vi "Load Image From Memory (Core).vi"(8 "error in (no error)":errorcluster, 9 "Transparency Threshold (127)":u8=127, 11 "Encoded Image":u8[](array[numeric])) -> (0 "error out":errorcluster, 2 "Image":T1)   [LabVIEW 2020, in "G-Image.lvlib"]
doc: "Decodes the byte array to a LabVIEW picture."
uses:
  G-Image.lvlib
  <vilib>/picture/picture.llb/imagedata.ctl
  <vilib>/Utility/file.llb/Application Directory.vi
  <vilib>/Utility/error.llb/Error Cluster From Error Code.vi
  lib/g_image_32.dll
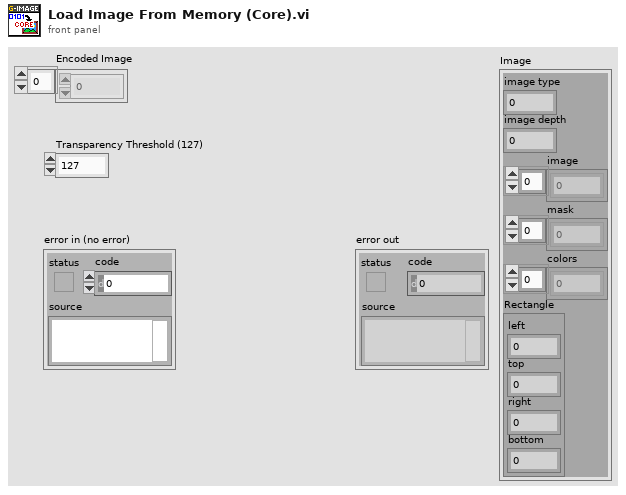
[diagram p1: front panel]
types:
  T1 = typedef "imagedata.ctl" = cluster{"image type":i32, "image depth":i32, "image":u8[], "mask":u8[], "colors":u32[], "Rectangle":cluster{"left":i16, "top":i16, "right":i16, "bottom":i16}}
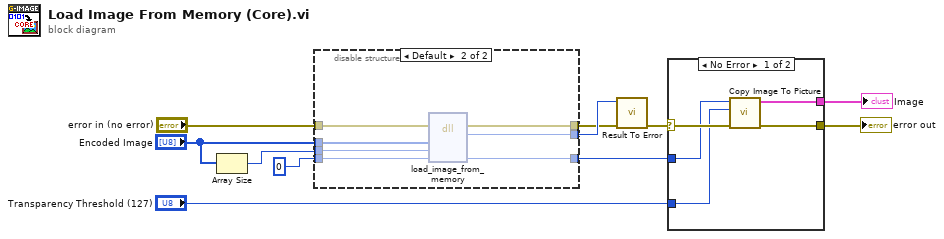
[diagram p0: block diagram]
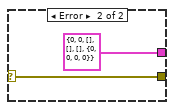
[diagram p2: hidden frame]
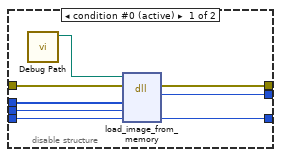
[diagram p3: hidden frame]
diagram:
  n1 = Array Size(array="Encoded Image") -> (size(s)=w2:i32)
  n2 = disable-structure shown="Default" {
    disable-tunnel: [w18 w26] -> w8
    disable-tunnel: "error in (no error)" -> [w17 w25]
    disable-tunnel: "Encoded Image" -> [w16 w24]
    disable-tunnel: [w15 w23] -> w9
    disable-tunnel: [w14 w21] -> w5
    disable-tunnel: i64 0 ("count") -> [w13 w22]
    disable-tunnel: w2 -> [w12 w20]
    frame condition #0 (active) {
      n3 = call "Debug Path.vi"() -> ("Debug Path"=w19:path)  [unwired: 11 in]
      n4 = dll-call lib="?" fn="load_image_from_memory"(path in=w19, error in=w17, "encoded_image"=w16, "encoded_image_size"=w12, "image_out"=w13) -> (error out=w18:errorcluster, "result"=w15:i32, "image_out"=w14:i64)  [unwired: 3 in, 1 out]
    }
    frame condition #1 {
      n5 = dll-call lib="C:/github/dataflowg/g-image/src/LabVIEW/G-Image/lib/g_image_*.*" fn="load_image_from_memory"(error in=w25, "encoded_image"=w24, "encoded_image_count"=w20, "image_out"=w22) -> (error out=w26:errorcluster, "result"=w23:i32, "image_out"=w21:i64)  [unwired: 4 in, 1 out]
    }
  }
  n6 = call "Result To Error.vi"("error in (no error)"=w8, "Result Code"=w9) -> ("error out"=w7:errorcluster)  [unwired: 9 in]
  n7 = case shown="No Error" w7 {
    selector: w7 -> [w31 w33]
    tunnel: [w29 w33] -> w11
    tunnel: w5 -> [w30 _]
    tunnel: [w28 T1 {"image type"=0, "image depth"=0, "image"=[], "mask"=[], "colors"=[], "Rectangle"={"left"=0, "top"=0, "right"=0, "bottom"=0}} ("Image")] -> w4
    tunnel: "Transparency Threshold (127)" -> [w27 _]
    frame No Error {
      n8 = call "Copy Image To Picture.vi"("error in (no error)"=w31, "Transparency Threshold (127)"=w27, "image_ptr"=w30) -> ("error out"=w29:errorcluster, "Picture"=w28:T1)  [unwired: 7 in]
    }
    frame Error {
    }
  }
  "error out" <- w11
  "Image" <- w4
